vi "SendLVEthIP_ExplicitMessage.vi"(8 "error in (no error)":errorcluster, 9 "value":i32, 10 "Motor Controller Parameter":T1, 11 "Refnum in":T2) -> (0 "error out":errorcluster, 3 "Refnum out":T2)   [LabVIEW 2022 SP3, in "Motor Controller.lvclass"]
uses:
  Motor Controller.lvclass
  <vilib>/ethernetip/ethernetip.llb/ethernetip.ctl
  Typedefs/Motor Controller Parameter-Set.ctl
  <vilib>/ethernetip/ethernetip.lvlib
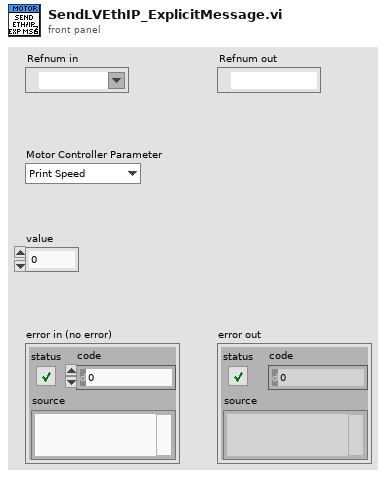
[diagram p1: front panel]
types:
  T1 = typedef "Motor Controller.lvclass/Motor Controller Parameter-Set.ctl" = enum16{"Print Speed", "Jog Speed", "PR Path", "Enable Servo", "Disable Servo", "Move Stage to Under PH1", "Move Stage to Under PH2", "Move Stage to Under PH3", "Move Stage to Under PH4", "Move Stage to Under PH5", "Move Stage to Under PH6", "Home Stage", "Return Stage to 0", "Print Stage", "Write Speed", "Write Index", "Stop Stage"}
  T2 = typedef "ethernetip.lvlib/ethernetip.ctl" = refnum<k21>
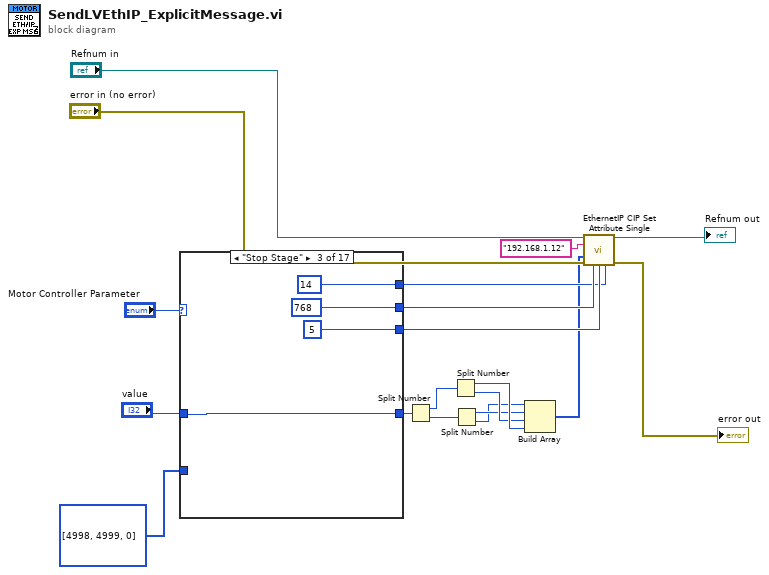
[diagram p0: block diagram]
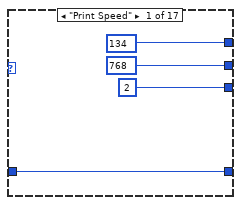
[diagram p2: hidden frame]
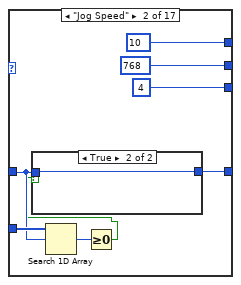
[diagram p3: hidden frame]
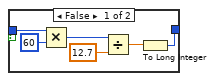
[diagram p4: hidden frame]
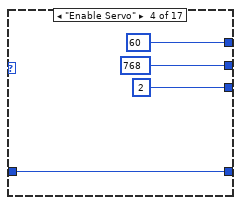
[diagram p5: hidden frame]
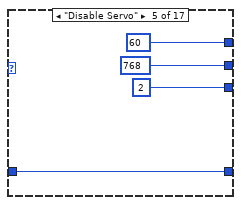
[diagram p6: hidden frame]
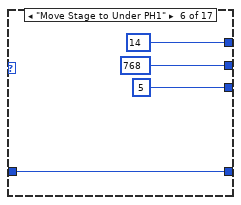
[diagram p7: hidden frame]
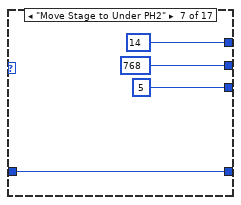
[diagram p8: hidden frame]
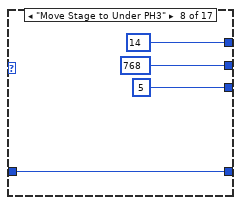
[diagram p9: hidden frame]
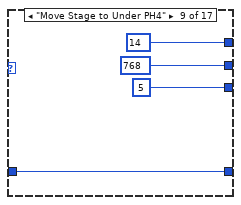
[diagram p10: hidden frame]
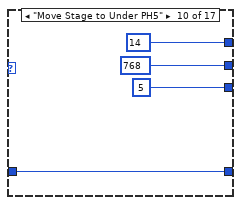
[diagram p11: hidden frame]
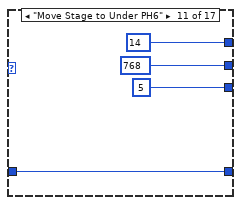
[diagram p12: hidden frame]
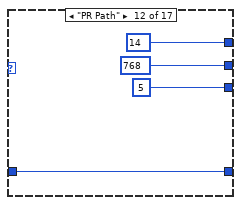
[diagram p13: hidden frame]
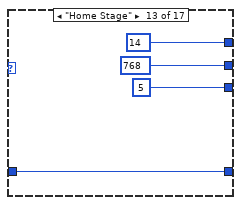
[diagram p14: hidden frame]
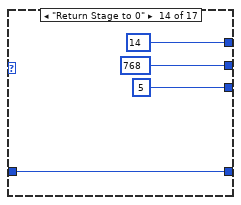
[diagram p15: hidden frame]
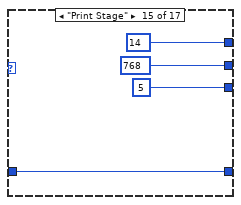
[diagram p16: hidden frame]
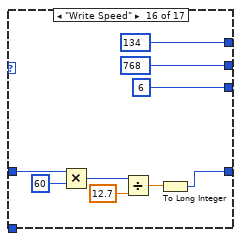
[diagram p17: hidden frame]
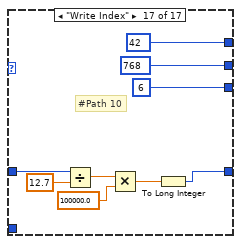
[diagram p18: hidden frame]
diagram:
  n1 = case shown="\"Stop Stage\"" "Motor Controller Parameter" {
    tunnel: [134 ("Attribute") 10 ("Attribute") 14 ("Attribute") 60 ("Attribute") 60 ("Attribute") 14 ("Attribute") 14 ("Attribute") 14 ("Attribute") 14 ("Attribute") 14 ("Attribute") 14 ("Attribute") 14 ("Attribute") 14 ("Attribute") 14 ("Attribute") 14 ("Attribute") 134 ("Attribute") 42 ("Attribute")] -> w14
    tunnel: [768 ("Class") 768 ("Class") 768 ("Class") 768 ("Class") 768 ("Class") 768 ("Class") 768 ("Class") 768 ("Class") 768 ("Class") 768 ("Class") 768 ("Class") 768 ("Class") 768 ("Class") 768 ("Class") 768 ("Class") 768 ("Class") 768 ("Class")] -> w17
    tunnel: [u32 2 ("assembly instance ID") u32 4 ("assembly instance ID") u32 5 ("assembly instance ID") u32 2 ("assembly instance ID") u32 2 ("assembly instance ID") u32 5 ("assembly instance ID") u32 5 ("assembly instance ID") u32 5 ("assembly instance ID") u32 5 ("assembly instance ID") u32 5 ("assembly instance ID") u32 5 ("assembly instance ID") u32 5 ("assembly instance ID") u32 5 ("assembly instance ID") u32 5 ("assembly instance ID") u32 5 ("assembly instance ID") u32 6 ("assembly instance ID") u32 6 ("assembly instance ID")] -> w16
    tunnel: [w20 w28 w39 w43 w47 w51 w55 w59 w63 w67 w71 w75 w79 w83 w87 w91 w100] -> w3
    tunnel: "value" -> [w20 w26 w39 w43 w47 w51 w55 w59 w63 w67 w71 w75 w79 w83 w87 w94 w102]
    tunnel: i32[] [4998, 4999, 0] -> [_ w27 _ _ _ _ _ _ _ _ _ _ _ _ _ _ _]
    frame "Print Speed" {
    }
    frame "Jog Speed" {
      n2 = Search 1D Array(1D array=w27, element=w26) -> (index of element=w25:i32)  [unwired: 1 in]
      n3 = Greater Or Equal To 0?(x=w25) -> (x >= 0?=w24:bool)
      n4 = case shown="True" w24 {
        tunnel: [w33 w38] -> w28
        tunnel: w26 -> [w32 w38]
        frame False {
          n5 = Multiply(x=w32, y=60 ("x")) -> (x*y=w35:i32)
          n6 = Divide(x=w35, y=12.7) -> (x/y=w34:dbl)
          n7 = To Long Integer(number=w34) -> (32bit integer=w33:i32)
        }
        frame True {
        }
      }
    }
    frame "Stop Stage" {
    }
    frame "Enable Servo" {
    }
    frame "Disable Servo" {
    }
    frame "Move Stage to Under PH1" {
    }
    frame "Move Stage to Under PH2" {
    }
    frame "Move Stage to Under PH3" {
    }
    frame "Move Stage to Under PH4" {
    }
    frame "Move Stage to Under PH5" {
    }
    frame "Move Stage to Under PH6" {
    }
    frame "PR Path" {
    }
    frame "Home Stage" {
    }
    frame "Return Stage to 0" {
    }
    frame "Print Stage" {
    }
    frame "Write Speed" {
      n8 = Multiply(x=w94, y=60 ("x")) -> (x*y=w93:i32)
      n9 = Divide(x=w93, y=12.7) -> (x/y=w92:dbl)
      n10 = To Long Integer(number=w92) -> (32bit integer=w91:i32)
    }
    frame "Write Index" {
      # "#Path 10"
      n11 = Divide(x=w102, y=12.7) -> (x/y=w105:dbl)
      n12 = Multiply(x=w105, y=100000.0 ("x")) -> (x*y=w101:dbl)
      n13 = To Long Integer(number=w101) -> (32bit integer=w100:i32)
    }
  }
  n14 = Split Number(x=w3) -> (hi(x)=w5:u16, lo(x)=w4:u16)
  n15 = Split Number(x=w5) -> (hi(x)=w9:u8, lo(x)=w8:u8)
  n16 = Split Number(x=w4) -> (hi(x)=w7:u8, lo(x)=w6:u8)
  n17 = Build Array(w6, w7, w8, w9) -> (w11:u8[])
  n18 = call <vilib>:"EthernetIP CIP Set Attribute Single.vi"("Session in"="Refnum in", "Network Path"="192.168.1.12", "Data"=w11, "error in"="error in (no error)", "Class"=w17, "Instance"=w16, "Attribute"=w14) -> ("Session out"=→"Refnum out":T2, "error out"=→"error out":errorcluster)  [unwired: 7 in]
